vi "set_target_resolution.vi"(8 "error in (no error)":errorcluster, 9 "y":i32, 10 "x":i32, 11 "MG090623BinningImageAssembler.lvclass in":refnum<class "ImageAssemblerMG090623Binning.lvclass">) -> (0 "error out":errorcluster, 3 "MG090623BinningImageAssembler.lvclass out":refnum<class "ImageAssemblerMG090623Binning.lvclass">)   [LabVIEW 2010, in "ImageAssemblerMG090623Binning.lvclass"]
uses:
  ImageAssemblerMG090623Binning.lvclass
  ImageAssemblerMG090623Binning.lvclass/ImageAssemblerMG090623Binning.ctl
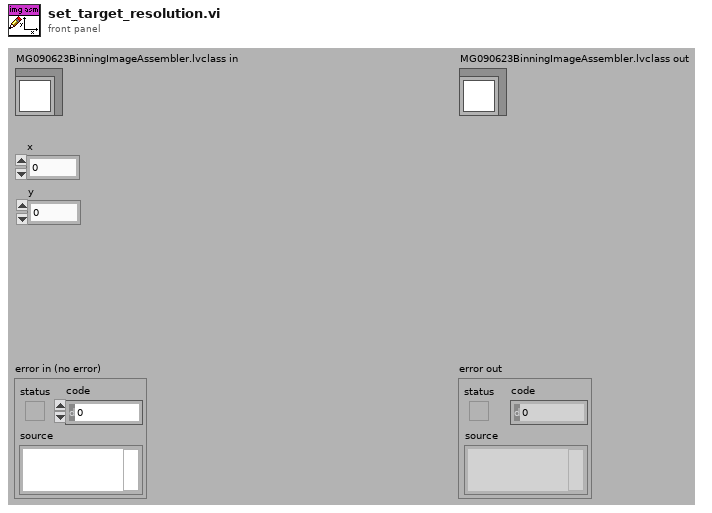
[diagram p1: front panel]
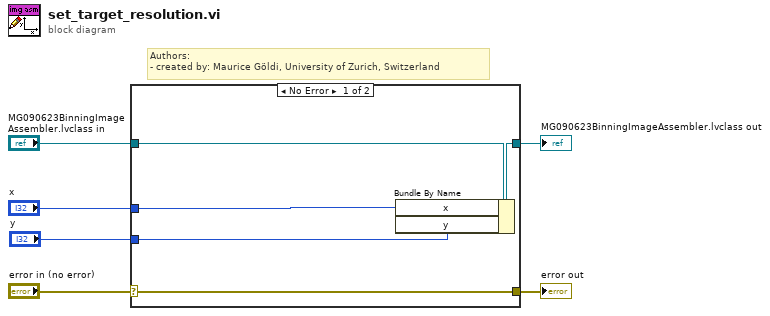
[diagram p0: block diagram]
diagram:
  # "Authors: \n- created by: Maurice Göldi, University of Zurich, Switzerland"
  n1 = case shown="No Error" "error in (no error)" {
    selector: "error in (no error)" -> [w11 w12]
    tunnel: [w11 w12] -> w5
    tunnel: [w9 w13] -> w3
    tunnel: "MG090623BinningImageAssembler.lvclass in" -> [w10 w13]
    tunnel: "x" -> [w8 _]
    tunnel: "y" -> [w7 _]
    frame No Error {
      n2 = Bundle By Name(cluster=w10, "x"=w8, "y"=w7) -> (w9:refnum<class "ImageAssemblerMG090623Binning.lvclass">)
    }
    frame Error {
    }
  }
  "error out" <- w5
  "MG090623BinningImageAssembler.lvclass out" <- w3
